vi "FKsolverbetter(SubVI).vi"(8 "q":dbl[](array[numeric]), 9 "Arm Lengths":cluster{"L 1":dbl, "L 2":dbl, "L 3":dbl}, 10 "empty picture":picture) -> (1 "end (2D)":cluster{"x":dbl, "y":dbl}, 2 "2D Picture 2":picture, 3 "Robot arm Final Position":cluster{"x2":dbl, "y2":dbl} {"x2" format="%#_6e"})   [LabVIEW 2024]
panel:
  out "chair end position":cluster{"X":dbl, "Y":dbl}={"X"=61.080020351084045, "Y"=-1.710100716628343}
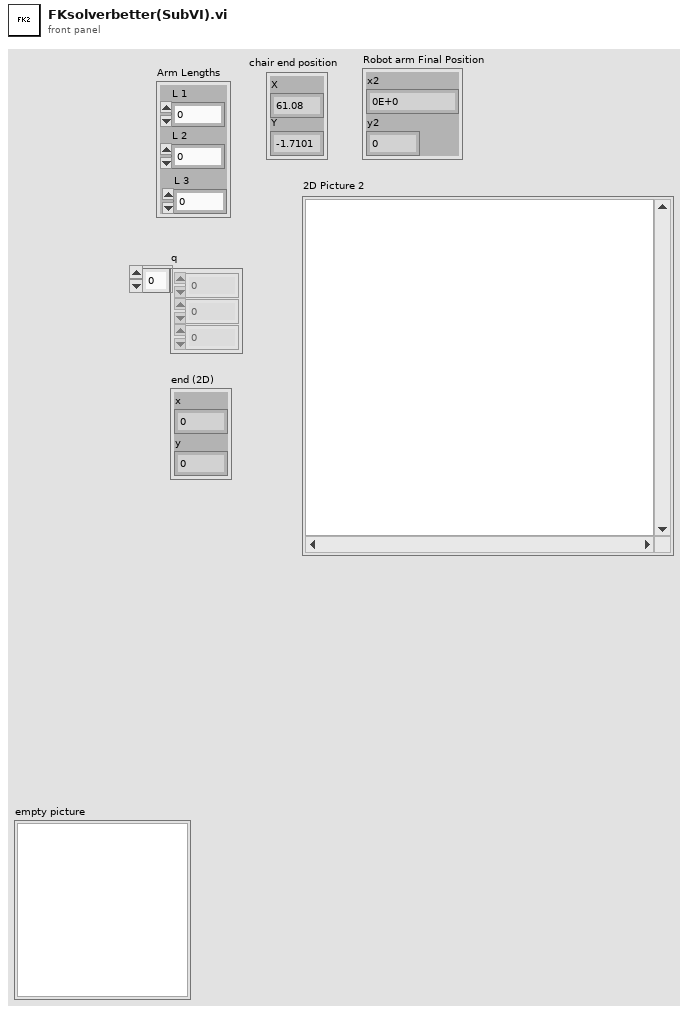
[diagram p1: front panel]
types:
  T1 = cluster{"Width":u16, "Style":enum32{"Solid", "Dash", "Dot", "DashDot", "DashDotDot"}}
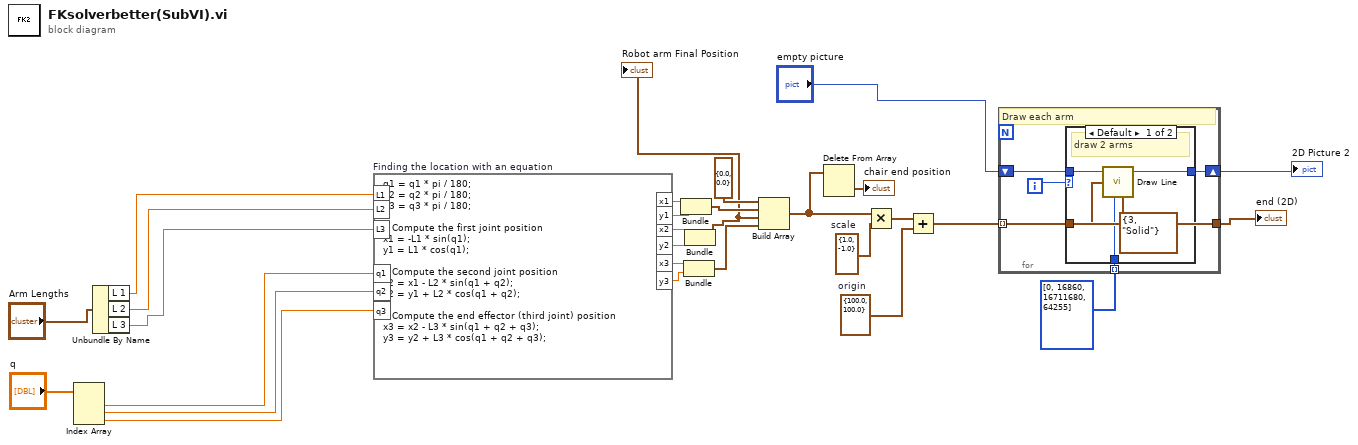
[diagram p0: block diagram]
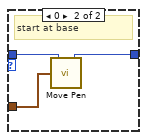
[diagram p2: hidden frame]
diagram:
  w21 = cluster{"x":dbl, "y":dbl} {"x"=1.0, "y"=-1.0}  # scale
  w22 = cluster{"x":dbl, "y":dbl} {"x"=100.0, "y"=100.0}  # origin
  n1 = Index Array(array="q") -> (element #1=w7:dbl, element #2=w6:dbl, element #3=w5:dbl)  [unwired: 3 in]
  n2 = Unbundle By Name("Arm Lengths") -> ("L 1"=w11:dbl, "L 2"=w10:dbl, "L 3"=w9:dbl)
  n3 = formula code="q1 = q1 * pi / 180; \nq2 = q2 * pi / 180;\nq3 = q3 * pi / 180;\n\n// Compute the first joint position\nx1 = -L1 * sin(q1);\ny1 = L1 * cos(q1);\n\n// Compute the second joint position\nx2 = x1 - L2 * sin(q1 + q2);\ny2 = y1 + L2 * cos(q1 + q2);\n\n// Compute the end effector (third joint) position\nx3 = x2 - L3 * sin(q1 + q2 + q3);\ny3 = y2 + L3 * cos(q1 + q2 + q3);" "Finding the location with an equation"("L1"=w11, "L2"=w10, "q2"=w6, "q1"=w7, "L3"=w9, "q3"=w5) -> ("x2"=w13:dbl, "y2"=w14:dbl, "x1"=w15:dbl, "y1"=w16:dbl, "x3"=w4:dbl, "y3"=w3:dbl)
  n4 = Bundle("x1"=w15, "y1"=w16) -> (w17:cluster{"x1":dbl, "y1":dbl})  [unwired: 1 in]
  n5 = Bundle("x3"=w4, "y3"=w3) -> (w2:cluster{"x3":dbl, "y3":dbl})  [unwired: 1 in]
  n6 = Bundle("x2"=w13, "y2"=w14) -> (w1:cluster{"x2":dbl, "y2":dbl})  [unwired: 1 in]
  "Robot arm Final Position" <- w1
  n7 = Build Array(cluster{"x":dbl, "y":dbl} {"x"=0.0, "y"=0.0} ("y"), w17, w1, w2) -> (w26:cluster{"x3":dbl, "y3":dbl}[])
  n8 = Delete From Array(array=w26) -> (deleted portion=→"chair end position":cluster{"x3":dbl, "y3":dbl})  [unwired: 2 in, 1 out]
  n9 = Multiply(x=w26, y=w21) -> (x*y=w23:cluster{dbl, dbl}[])
  n10 = Add(x=w23, y=w22) -> (x+y=w24:cluster{dbl, dbl}[])
  n11 = for {
    shift-right: [w31] -> w19
    shift-left: "empty picture" -> [w32]
    tunnel: u32[] [0, 16860, 16711680, 64255] -> [w30] mode=indexing
    tunnel: w24 -> [w29] mode=indexing
    tunnel: [w29] -> w27
    i -> [w33]
    # "Draw each arm"
    n12 = case shown="Default" w33 {
      tunnel: w32 -> [w38 w41]
      tunnel: [w37 w40] -> w31
      tunnel: w29 -> [w36 w39]
      tunnel: w30 -> [w35 _]
      frame Default {
        # "draw 2 arms"
        n13 = call <vilib>:"Draw Line.vi"("picture"=w38, "end point"=w36, "color(black)"=w35, "pen"=T1 {"Width"=3, "Style"=enum."Solid"}) -> ("new picture"=w37:picture)  [unwired: 5 in]
      }
      frame 0 {
        # "start at base"
        n14 = call <vilib>:"Move Pen.vi"("new position"=w39, "picture"=w41) -> ("new picture"=w40:picture)  [unwired: 3 in]
      }
    }
  }
  "2D Picture 2" <- w19
  "end (2D)" <- w27
